vi "Device Count.vi"(11 "VoiceMeeterRemote in":refnum<class "VoiceMeeterRemote.lvclass">) -> (2 "Device Count":i32, 3 "VoiceMeeterRemote out":refnum<class "VoiceMeeterRemote.lvclass">)   [LabVIEW 2022 SP3, in "VoiceMeeterRemote.lvlib" / "VoiceMeeterRemote.lvclass"]
doc: "Returns the total number of devices routable by Voicemeeter including both inputs and outputs."
uses:
  VoiceMeeterRemote.lvclass
  VoiceMeeterRemote.lvclass/VoiceMeeterRemote.ctl
  VoiceMeeterRemote.lvlib
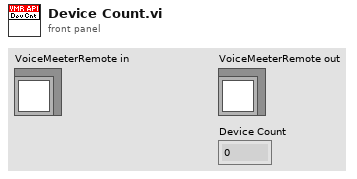
[diagram p1: front panel]
types:
  T1 = typedef "VoiceMeeterRemote.lvlib/Voicemeeter Type.ctl" = enum16{"Unknown", "Voicemeeter", "Banana", "Potato", "Potato x64"}
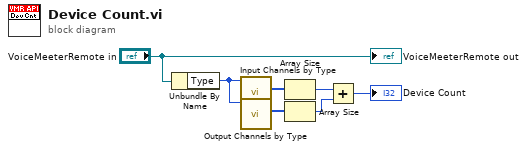
[diagram p0: block diagram]
diagram:
  n1 = Unbundle By Name("VoiceMeeterRemote in") -> ("Type"=w7:T1)
  n2 = call "Input Channels by Type.vi"("Voicemeeter Type"=w7) -> ("Channel Count"=w4:i32[])  [unwired: 10 in]
  n3 = call "Output Channels by Type.vi"("Voicemeeter Type"=w7) -> ("Channel Count"=w5:i32[])  [unwired: 10 in]
  n4 = Array Size(array=w4) -> (size(s)=w3:i32)
  n5 = Array Size(array=w5) -> (size(s)=w2:i32)
  n6 = Add(x=w3, y=w2) -> (x+y=→"Device Count":i32)
  "VoiceMeeterRemote out" <- "VoiceMeeterRemote in"
